vi "Check Fault.vi"(11 "Array":bool[](array[boolean])) -> (2 "Fault Index":i32, 3 "Fault?":bool)   [LabVIEW 2014]
uses:
  RT Tags.vi
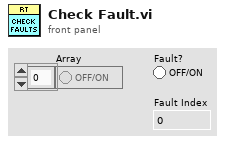
[diagram p1: front panel]
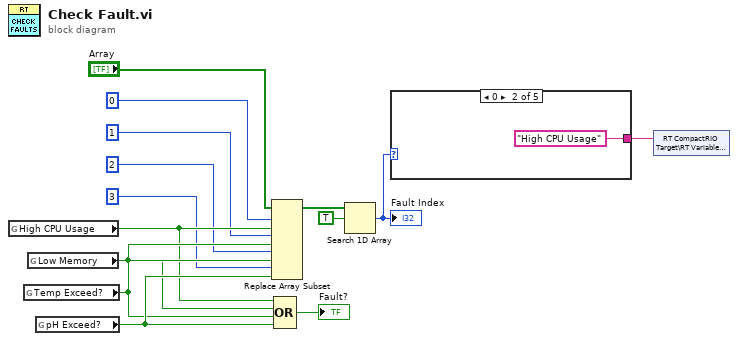
[diagram p0: block diagram]
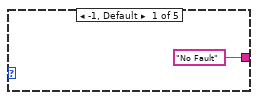
[diagram p2: hidden frame]
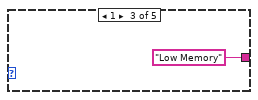
[diagram p3: hidden frame]
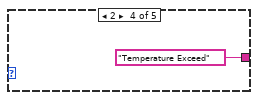
[diagram p4: hidden frame]
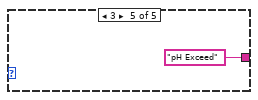
[diagram p5: hidden frame]
diagram:
  n1 = global read "RT Tags.vi" "High CPU Usage"() -> (w6:bool)
  n2 = global read "RT Tags.vi" "Temp Exceed?"() -> (w8:bool)
  n3 = global read "RT Tags.vi" "Low Memory"() -> (w7:bool)
  n4 = global read "RT Tags.vi" "pH Exceed?"() -> (w9:bool)
  n5 = Replace Array Subset(array="Array", new element #1=w6, index #1=0 ("index"), new element #2=w7, index #2=1 ("index"), new element #3=w8, index #3=2 ("index"), new element #4=w9, index #4=3 ("index")) -> (w11:bool[])
  n6 = Compound Arithmetic op=OR(w6, w7, w8, w9) -> (→"Fault?":bool)
  n7 = Search 1D Array(1D array=w11, element=TRUE) -> (index of element=w13:i32)  [unwired: 1 in]
  "Fault Index" <- w13
  n8 = case shown="0" w13 {
    tunnel: ["No Fault" "High CPU Usage" "Low Memory" "Temperature Exceed" "pH Exceed"] -> w14
    frame -1, Default {
    }
    frame 0 {
    }
    frame 1 {
    }
    frame 2 {
    }
    frame 3 {
    }
  }
  n9 = shared-variable "RT CompactRIO Target\\RT Variables.lvlib\\Faults"(w14) -> ()  [unwired: 1 in, 1 out]
